vi "MKH.vi"() -> ()   [LabVIEW 2015]
uses:
  Control MKH.ctl
  Control MKH2.ctl
panel:
  in  "NEXT":bool caption="START/STOP"
  in  "stop 2":bool
  out "Count":i32=100
  out "State":string
  out "HIJAU 2":bool=TRUE
  out "MERAH 2":bool=TRUE
  out "KUNING 2":bool=TRUE
  out "\\":bool=TRUE
  out "?":bool=TRUE
  out "?":bool=TRUE
  in  "START/STOP":bool
  out "MERAH":bool=TRUE
  out "HIJAU":bool=TRUE
  out "KUNING":bool=TRUE
  out "String 2":string
  in  "stop":bool
  out "x-1":i32
  out "STATE":string="MERAH"
  out "COUNT":i32
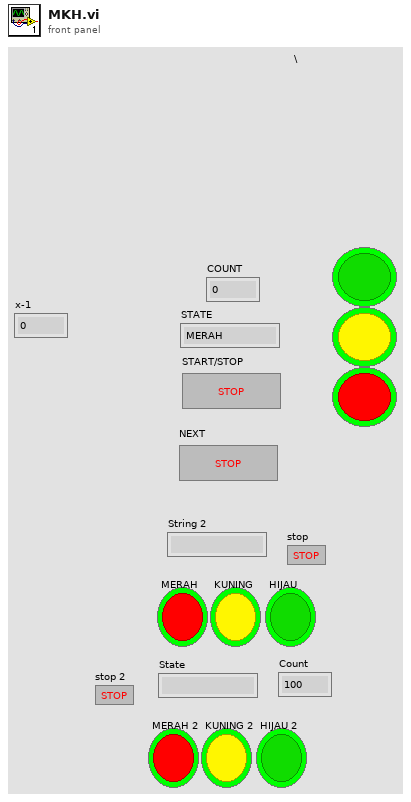
[diagram p1: front panel]
types:
  T1 = typedef "Control MKH2.ctl" = enum16{"Hi", "Ku", "Me", "Stop"}
  T2 = typedef "Control MKH.ctl" = enum16{"START", "INITIALIZE", "MERAH", "KUNING", "HIJAU", "CONTINUE??", "STOP", ""}
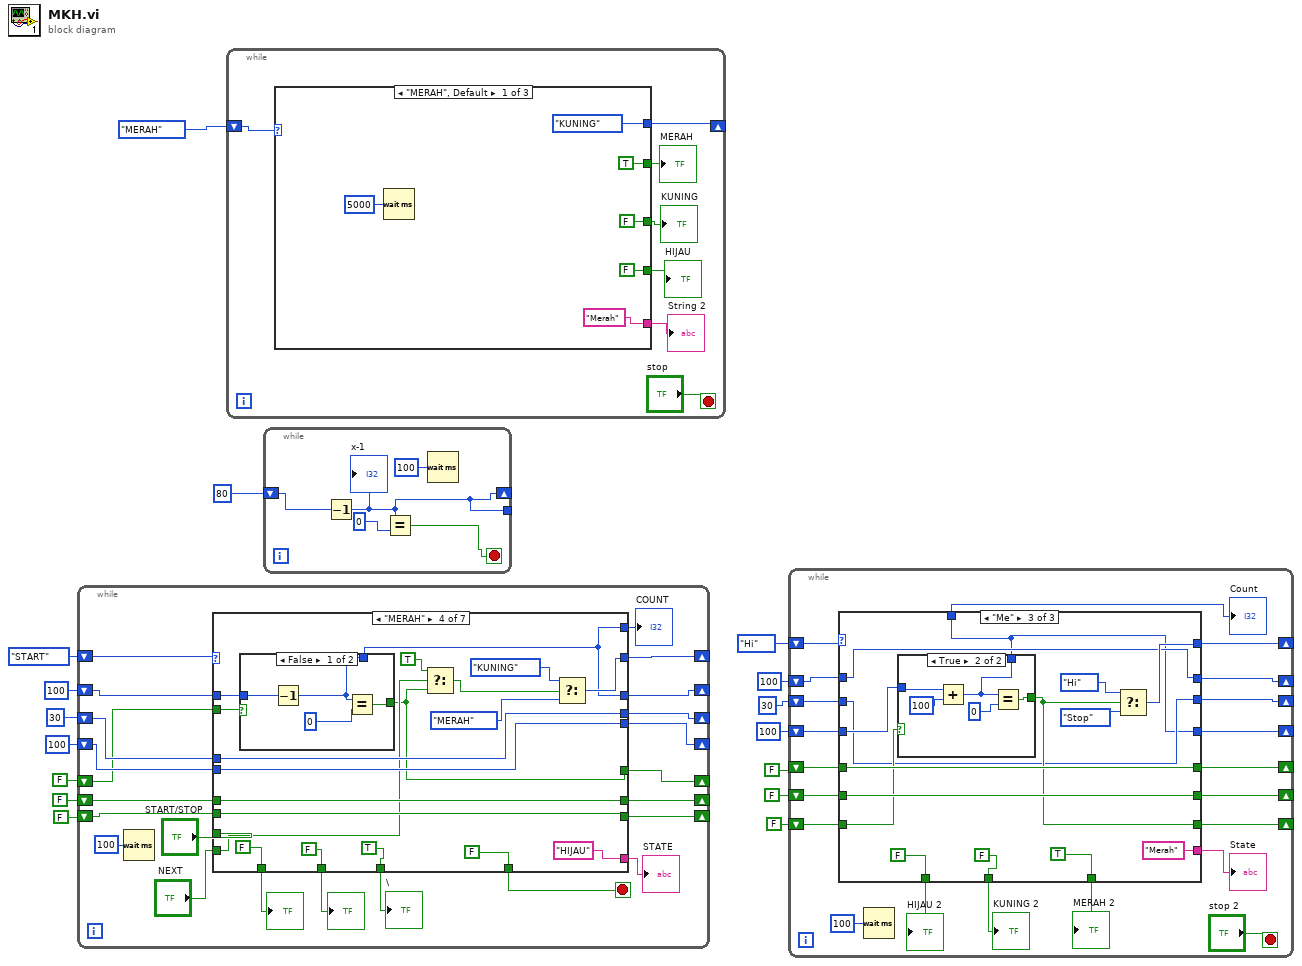
[diagram p0: block diagram]
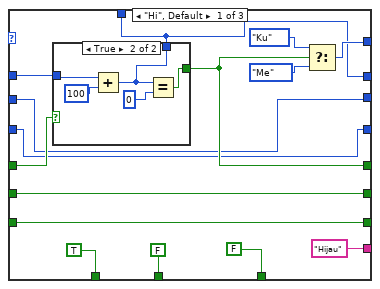
[diagram p2: hidden frame]
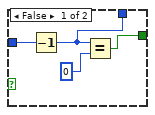
[diagram p3: hidden frame]
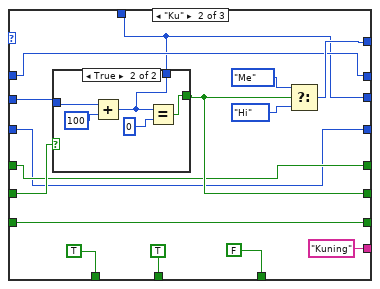
[diagram p4: hidden frame]
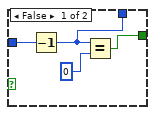
[diagram p5: hidden frame]
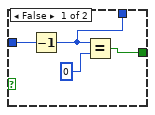
[diagram p6: hidden frame]
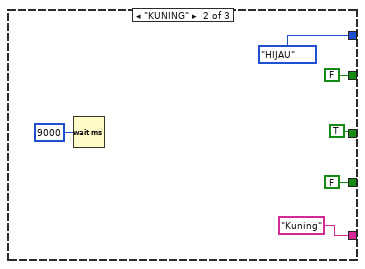
[diagram p7: hidden frame]
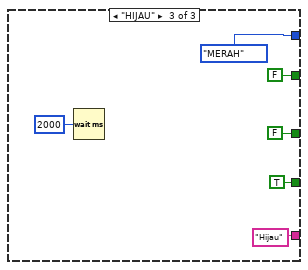
[diagram p8: hidden frame]
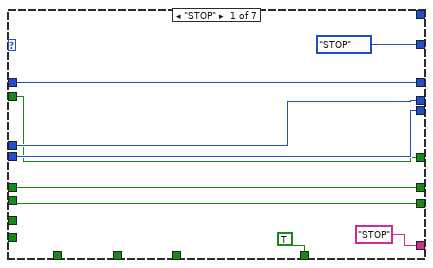
[diagram p9: hidden frame]
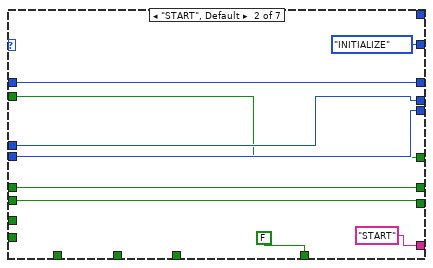
[diagram p10: hidden frame]
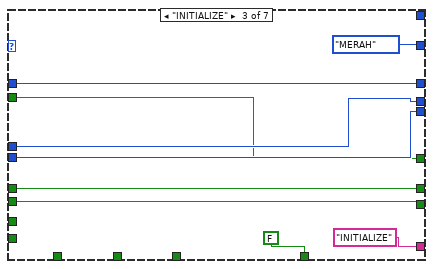
[diagram p11: hidden frame]
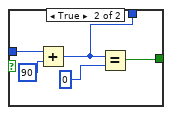
[diagram p12: hidden frame]
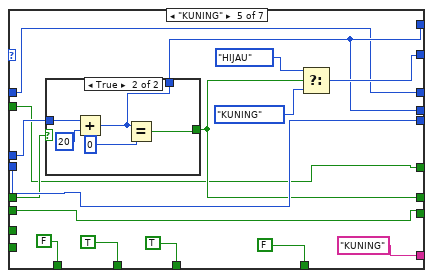
[diagram p13: hidden frame]
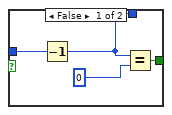
[diagram p14: hidden frame]
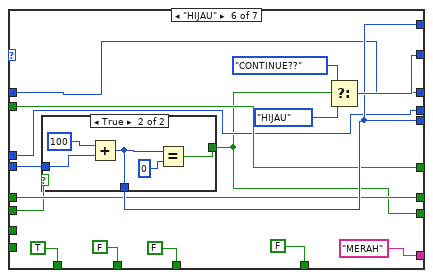
[diagram p15: hidden frame]
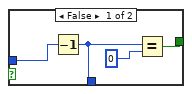
[diagram p16: hidden frame]
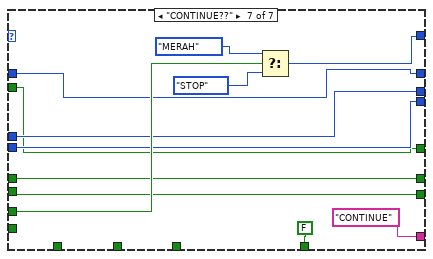
[diagram p17: hidden frame]
diagram:
  n1 = while {
    shift-right: [w38] -> _
    shift-left: Control_MKH."START" -> [w39]
    shift-right: [w31] -> _
    shift-left: 100 -> [w33]
    shift-right: [w30] -> _
    shift-left: 30 -> [w29]
    shift-right: [w27] -> _
    shift-left: 100 -> [w28]
    shift-right: [w25] -> _
    shift-left: FALSE -> [w26]
    shift-right: [w23] -> _
    shift-left: FALSE -> [w24]
    shift-right: [w21] -> _
    shift-left: FALSE -> [w22]
    stop <- w37 stop-if-true
    n2 = Wait (ms)(milliseconds to wait=u32 100) -> ()  [unwired: 1 out]
    n3 = case shown="\"MERAH\"" w39 {
      tunnel: [Control_MKH."STOP" Control_MKH."INITIALIZE" Control_MKH."MERAH" w83 w106 w132 w156] -> w38
      tunnel: [TRUE FALSE FALSE FALSE FALSE FALSE FALSE] -> w37
      tunnel: ["STOP" "START" "INITIALIZE" "HIJAU" "KUNING" "MERAH" "CONTINUE"] -> w36
      tunnel: "START/STOP" -> [_ _ _ _ _ _ w154]
      tunnel: [_ _ _ FALSE FALSE TRUE _] -> w20
      tunnel: [_ _ _ FALSE TRUE FALSE _] -> w19
      tunnel: [_ _ _ TRUE TRUE FALSE _] -> w18
      tunnel: w33 -> [w45 w54 w64 w80 w99 w129 w150]
      tunnel: [_ _ _ w79 w100 w130 _] -> w32
      tunnel: [w45 w54 w64 w79 w99 w129 w150] -> w31
      tunnel: [w44 w53 w63 w78 w100 w125 w149] -> w30
      tunnel: w29 -> [w44 w53 w63 w78 w104 w125 w149]
      tunnel: w28 -> [w43 w52 w62 w77 w105 w131 w148]
      tunnel: [w43 w52 w62 w77 w105 w130 w148] -> w27
      tunnel: w26 -> [w42 w51 w61 w76 w101 w128 w147]
      tunnel: [w42 w51 w61 w67 w101 w128 w147] -> w25
      tunnel: [w41 w50 w60 w75 w103 w127 w146] -> w23
      tunnel: w24 -> [w41 w50 w60 w75 w102 w127 w146]
      tunnel: w22 -> [w40 w49 w59 w74 w98 w126 w145]
      tunnel: [w40 w49 w59 w74 w98 w123 w145] -> w21
      tunnel: "NEXT" -> [_ _ _ w70 _ _ _]
      frame "STOP" {
      }
      frame "START", Default {
      }
      frame "INITIALIZE" {
      }
      frame "MERAH" {
        n4 = case shown="False" w76 {
          tunnel: [w89 w91] -> w67
          tunnel: w80 -> [w88 w94]
          tunnel: [w87 w90] -> w79
          frame False {
            n5 = Decrement(x=w88) -> (x-1=w87:i32)
            n6 = Equal?(x=w87, y=0) -> (x = y?=w89:bool)
          }
          frame True {
            n7 = Add(x=w94, y=90) -> (x+y=w90:i32)
            n8 = Equal?(x=w90, y=0) -> (x = y?=w91:bool)
          }
        }
        n9 = Select(t=TRUE, s=w70, f=w67) -> (s? t:f=w68:bool)
        n10 = Select(t=Control_MKH."KUNING", s=w68, f=Control_MKH."MERAH") -> (s? t:f=w83:T2)
      }
      frame "KUNING" {
        n11 = case shown="True" w102 {
          tunnel: [w114 w117] -> w100
          tunnel: w104 -> [w112 w116]
          tunnel: [w111 w115] -> w103
          frame False {
            n12 = Decrement(x=w112) -> (x-1=w114:i32)
            n13 = Equal?(x=w114, y=0) -> (x = y?=w111:bool)
          }
          frame True {
            n14 = Add(x=w116, y=20) -> (x+y=w117:i32)
            n15 = Equal?(x=w117, y=0) -> (x = y?=w115:bool)
          }
        }
        n16 = Select(t=Control_MKH."HIJAU", s=w103, f=Control_MKH."KUNING") -> (s? t:f=w106:T2)
      }
      frame "HIJAU" {
        n17 = case shown="True" w126 {
          tunnel: w131 -> [w138 w144]
          tunnel: [w137 w140] -> w123
          tunnel: [w136 w142] -> w130
          frame False {
            n18 = Decrement(x=w138) -> (x-1=w136:i32)
            n19 = Equal?(x=w136, y=0) -> (x = y?=w137:bool)
          }
          frame True {
            n20 = Add(x=100, y=w144) -> (x+y=w142:i32)
            n21 = Equal?(x=w142, y=0) -> (x = y?=w140:bool)
          }
        }
        n22 = Select(t=Control_MKH."CONTINUE??", s=w123, f=Control_MKH."HIJAU") -> (s? t:f=w132:T2)
      }
      frame "CONTINUE??" {
        n23 = Select(t=Control_MKH."MERAH", s=w154, f=Control_MKH."STOP") -> (s? t:f=w156:T2)
      }
    }
    "STATE" <- w36
    "COUNT" <- w32
    "?" <- w20
    "?" <- w19
    "\\" <- w18
  }
  n24 = while {
    shift-right: [w162] -> _
    shift-left: Control_MKH."MERAH" -> [w163]
    stop <- "stop" stop-if-true
    n25 = case shown="\"MERAH\", Default" w163 {
      tunnel: [Control_MKH."KUNING" Control_MKH."HIJAU" Control_MKH."MERAH"] -> w162
      tunnel: ["Merah" "Kuning" "Hijau"] -> w160
      tunnel: [FALSE FALSE TRUE] -> w159
      tunnel: [TRUE FALSE FALSE] -> w158
      tunnel: [FALSE TRUE FALSE] -> w157
      frame "MERAH", Default {
        n26 = Wait (ms)(milliseconds to wait=u32 5000) -> ()  [unwired: 1 out]
      }
      frame "KUNING" {
        n27 = Wait (ms)(milliseconds to wait=u32 9000) -> ()  [unwired: 1 out]
      }
      frame "HIJAU" {
        n28 = Wait (ms)(milliseconds to wait=u32 2000) -> ()  [unwired: 1 out]
      }
    }
    "String 2" <- w160
    "HIJAU" <- w159
    "MERAH" <- w158
    "KUNING" <- w157
  }
  n29 = while {
    shift-right: [w183] -> _
    shift-left: 80 -> [w185]
    tunnel: [w183] -> _
    stop <- w184 stop-if-true
    n30 = Decrement(x=w185) -> (x-1=w183:i32)
    "x-1" <- w183
    n31 = Equal?(x=w183, y=0) -> (x = y?=w184:bool)
    n32 = Wait (ms)(milliseconds to wait=u32 100) -> ()  [unwired: 1 out]
  }
  n33 = while {
    shift-right: [w205] -> _
    shift-left: Control_MKH2."Hi" -> [w204]
    shift-right: [w199] -> _
    shift-left: 100 -> [w203]
    shift-right: [w187] -> _
    shift-left: 30 -> [w198]
    shift-right: [w189] -> _
    shift-left: 100 -> [w188]
    shift-right: [w202] -> _
    shift-left: FALSE -> [w201]
    shift-right: [w196] -> _
    shift-left: FALSE -> [w195]
    shift-right: [w194] -> _
    shift-left: FALSE -> [w193]
    stop <- "stop 2" stop-if-true
    n34 = case shown="\"Me\"" w204 {
      tunnel: [w222 w243 w261] -> w205
      tunnel: w203 -> [w221 w242 w260]
      tunnel: [w211 w239 w267] -> w202
      tunnel: w201 -> [w218 w239 w267]
      tunnel: [w208 w232 w256] -> w200
      tunnel: [w208 w242 w260] -> w199
      tunnel: w198 -> [w209 w246 w257]
      tunnel: ["Hijau" "Kuning" "Merah"] -> w197
      tunnel: [w216 w240 w266] -> w196
      tunnel: w195 -> [w216 w241 w266]
      tunnel: [w215 w237 w259] -> w194
      tunnel: w193 -> [w215 w237 w262]
      tunnel: [TRUE TRUE FALSE] -> w192
      tunnel: [FALSE TRUE FALSE] -> w191
      tunnel: [FALSE FALSE TRUE] -> w190
      tunnel: [w210 w238 w256] -> w189
      tunnel: w188 -> [w210 w238 w263]
      tunnel: [w209 w232 w257] -> w187
      frame "Hi", Default {
        n35 = case shown="True" w218 {
          tunnel: w221 -> [w226 w231]
          tunnel: [w224 w228] -> w211
          tunnel: [w223 w227] -> w208
          frame False {
            n36 = Decrement(x=w226) -> (x-1=w223:i32)
            n37 = Equal?(x=w223, y=0) -> (x = y?=w224:bool)
          }
          frame True {
            n38 = Add(x=w231, y=100) -> (x+y=w227:i32)
            n39 = Equal?(x=w227, y=0) -> (x = y?=w228:bool)
          }
        }
        n40 = Select(t=Control_MKH2."Ku", s=w211, f=Control_MKH2."Me") -> (s? t:f=w222:T1)
      }
      frame "Ku" {
        n41 = case shown="True" w241 {
          tunnel: w246 -> [w250 w255]
          tunnel: [w248 w252] -> w240
          tunnel: [w247 w251] -> w232
          frame False {
            n42 = Decrement(x=w250) -> (x-1=w247:i32)
            n43 = Equal?(x=w247, y=0) -> (x = y?=w248:bool)
          }
          frame True {
            n44 = Add(x=w255, y=100) -> (x+y=w251:i32)
            n45 = Equal?(x=w251, y=0) -> (x = y?=w252:bool)
          }
        }
        n46 = Select(t=Control_MKH2."Me", s=w240, f=Control_MKH2."Hi") -> (s? t:f=w243:T1)
      }
      frame "Me" {
        n47 = case shown="True" w262 {
          tunnel: w263 -> [w274 w279]
          tunnel: [w272 w276] -> w259
          tunnel: [w271 w275] -> w256
          frame False {
            n48 = Decrement(x=w274) -> (x-1=w271:i32)
            n49 = Equal?(x=w271, y=0) -> (x = y?=w272:bool)
          }
          frame True {
            n50 = Add(x=w279, y=100) -> (x+y=w275:i32)
            n51 = Equal?(x=w275, y=0) -> (x = y?=w276:bool)
          }
        }
        n52 = Select(t=Control_MKH2."Hi", s=w259, f=Control_MKH2."Stop") -> (s? t:f=w261:T1)
      }
    }
    "State" <- w197
    "HIJAU 2" <- w192
    "MERAH 2" <- w190
    "KUNING 2" <- w191
    "Count" <- w200
    n53 = Wait (ms)(milliseconds to wait=u32 100) -> ()  [unwired: 1 out]
  }
